vi "EME 185B LabVIEW (arbirary signal).vi"() -> ()   [LabVIEW 2025]
uses:
  <vilib>/Utility/file.llb/Write Delimited Spreadsheet (string).vi
  <vilib>/Utility/file.llb/Write Delimited Spreadsheet (DBL).vi
panel:
  out "Waveform Graph":dynamicdata(graph)
  in  "stop":bool=TRUE
  out "XY Graph":cluster{dbl[], dbl[]}(graph)
  out "Elapsed Time (sec)":dbl
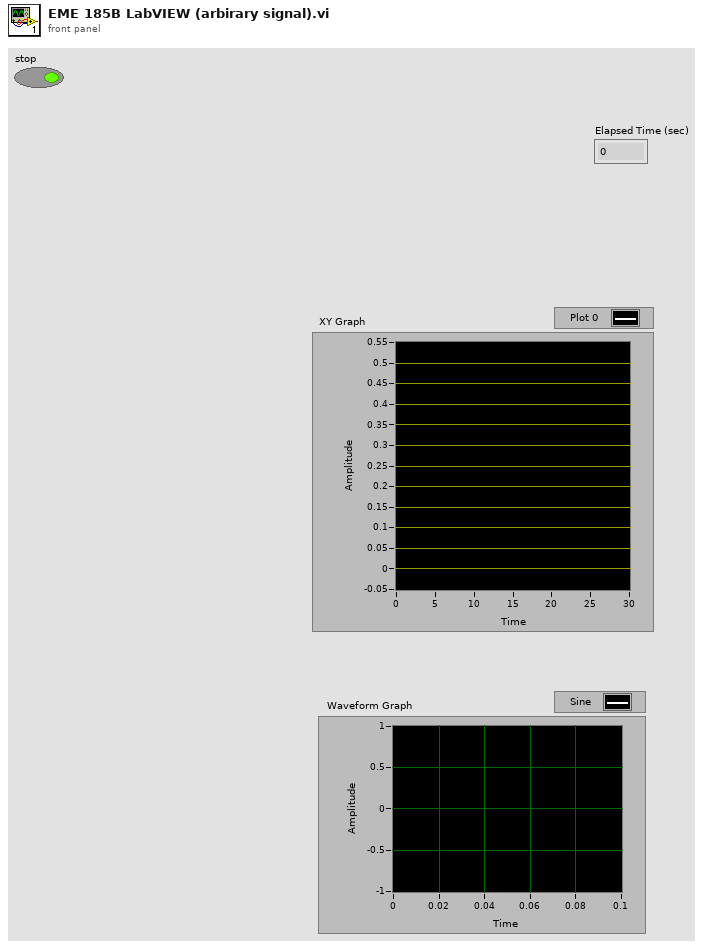
[diagram p1: front panel]
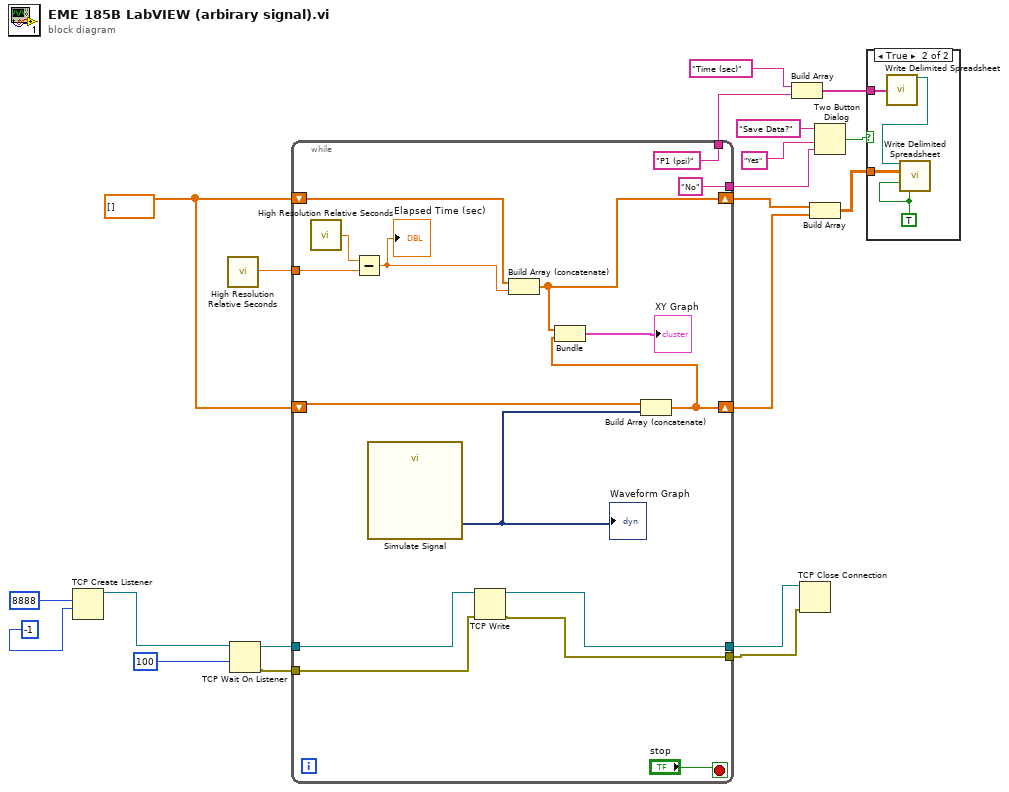
[diagram p0: block diagram]
diagram:
  w16 = dbl[] []
  n1 = TCP Create Listener(9:-1 ("timeout ms (25000)"), 10:u16 8888 ("port")) -> (3:w5:refnum<k5>)  [unwired: 3 in, 2 out]
  n2 = call <vilib>:"High Resolution Relative Seconds.vi"() -> ("relative seconds"=w20:dbl)
  n3 = TCP Wait On Listener(9:100 ("timeout ms (wait forever: -1)"), 11:w5) -> (0:w2:errorcluster, 4:w7:refnum<k5>)  [unwired: 2 in, 3 out]
  n4 = while {
    tunnel: w20 -> [w34]
    shift-right: [w30] -> w19
    shift-left: w16 -> [w32]
    shift-right: [w29] -> w18
    shift-left: w16 -> [w31]
    tunnel: ["P1 (psi)"] -> w13
    tunnel: ["No" ("F button name (\"Cancel\")")] -> w9
    tunnel: w7 -> [w25]
    tunnel: [w24] -> w6
    tunnel: w2 -> [w22]
    tunnel: [w21] -> w1
    stop <- "stop" stop-if-true
    n5 = call <vilib>:"High Resolution Relative Seconds.vi"() -> ("relative seconds"=w35:dbl)
    n6 = Subtract(x=w35, y=w34) -> (x-y=w33:dbl)
    "Elapsed Time (sec)" <- w33
    n7 = call "Simulate Signal"() -> ("Sine"=w23:dynamicdata)  [unwired: 14 in, 1 out]
    "Waveform Graph" <- w23
    n8 = TCP Write(connection ID=w25, error in (no error)=w22) -> (connection ID out=w24:refnum<k5>, error out=w21:errorcluster)  [unwired: 2 in, 1 out]
    n9 = Build Array (concatenate)(w32, w33) -> (w30:dbl[])
    n10 = Build Array (concatenate)(w31, w23) -> (w29:dbl[])
    n11 = Bundle(w30, w29) -> (→"XY Graph":cluster{dbl[], dbl[]})  [unwired: 1 in]
  }
  n12 = Build Array("Time (sec)", w13) -> (w14:string[])
  n13 = TCP Close Connection(connection ID=w6, error in (no error)=w1) -> ()  [unwired: 1 in, 2 out]
  n14 = Build Array(w19, w18) -> (w17:dbl[][])
  n15 = Two Button Dialog(message="Save Data?", 1:w9, 2:"Yes" ("T button name (\"OK\")")) -> (T button?=w12:bool)
  n16 = case shown="True" w12 {
    tunnel: w17 -> [_ w40]
    tunnel: w14 -> [_ w39]
    frame False {
    }
    frame True {
      w37 = TRUE ("transpose? (no:F)")
      n17 = call-poly <vilib>:"Write Delimited Spreadsheet.vi"("1D data"=w39) -> ("new file path (Not A Path if cancelled)"=w38:path)  [unwired: 13 in, 1 out]
      n18 = call-poly <vilib>:"Write Delimited Spreadsheet.vi"("file path (dialog if empty)"=w38, "2D data"=w40, "append to file? (new file:F)"=w37, "transpose? (no:F)"=w37) -> ()  [unwired: 10 in, 2 out]
    }
  }
